vi "CreateFile_in_a_folder_with_date_stamp.vi"(0 "Operator's Name":string, 1 "Data output folder":string="E:\\Ankit\\") -> (2 "filename":string, 3 "String":string, 4 "Path":path)   [LabVIEW 2013]
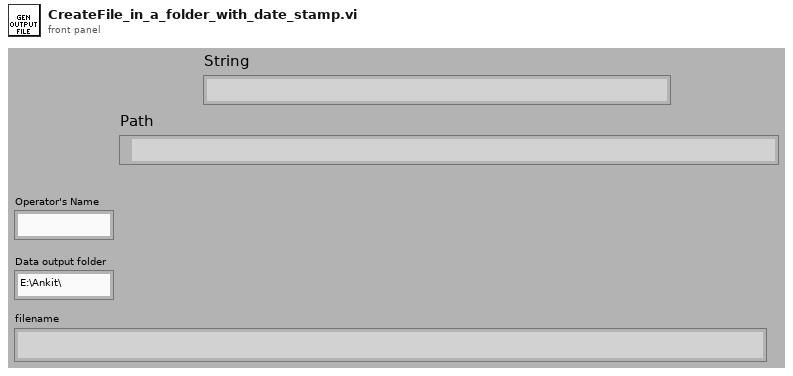
[diagram p1: front panel]
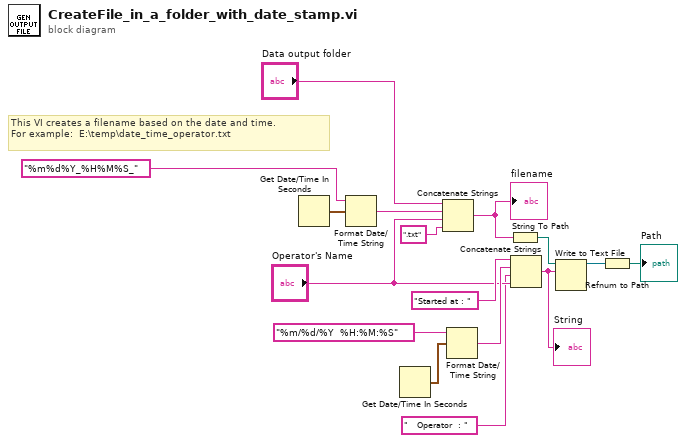
[diagram p0: block diagram]
diagram:
  # "This VI creates a filename based on the date and time.\nFor example:  E:\\temp\\date_time_operator.txt"
  n1 = Get Date/Time In Seconds() -> (seconds since 1Jan1904=w14:timestamp)
  n2 = Format Date/Time String(time format string (%c)="%m%d%Y_%H%M%S_", seconds (now)=w14) -> (date/time string=w9:string)  [unwired: 1 out]
  n3 = Get Date/Time In Seconds() -> (seconds since 1Jan1904=w8:timestamp)
  n4 = Concatenate Strings("Data output folder", w9, "Operator's Name", ".txt" ("string")) -> (w16:string)
  "filename" <- w16
  n5 = Format Date/Time String(time format string (%c)="%m/%d/%Y  %H:%M:%S", seconds (now)=w8) -> (date/time string=w6:string)  [unwired: 1 out]
  n6 = String To Path(string=w16) -> (path=w13:path)
  n7 = Concatenate Strings("Started at : " ("text"), w6, "   Operator  : " ("text"), "Operator's Name") -> (w1:string)
  "String" <- w1
  n8 = Write to Text File(file (use dialog)=w13, text=w1) -> (refnum out=w3:refnum<file>)  [unwired: 1 in, 3 out]
  n9 = Refnum to Path(1:w3) -> (0:→"Path":path)
